vi "Task7_with_case.vi"() -> ()   [LabVIEW 2017]
panel:
  out "String":string
  out "Binary":i8 format="%b"
  out "Decimal":string
  out "Octal":string
  out "Hexadecimal":string
  in  "Array":bool[](array[boolean])
  in  "0 - binary, 1 - octal, 2 - decimal, 3 - hexadecimal":u8(knob) scale=0.0..3.0
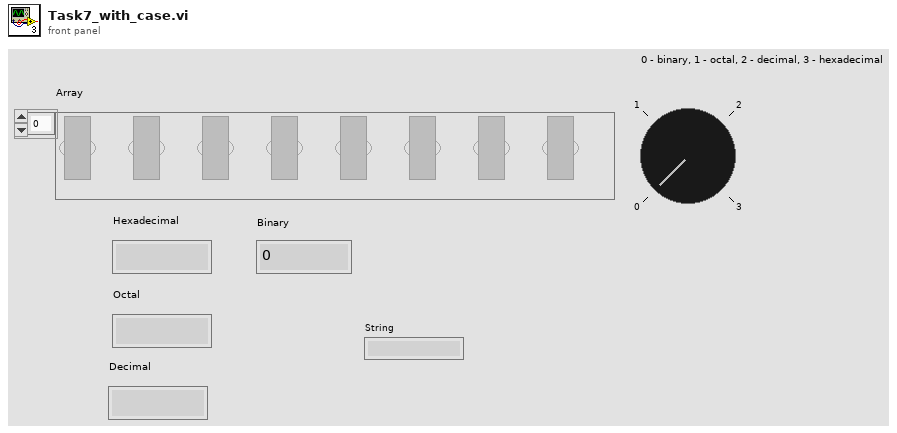
[diagram p1: front panel]
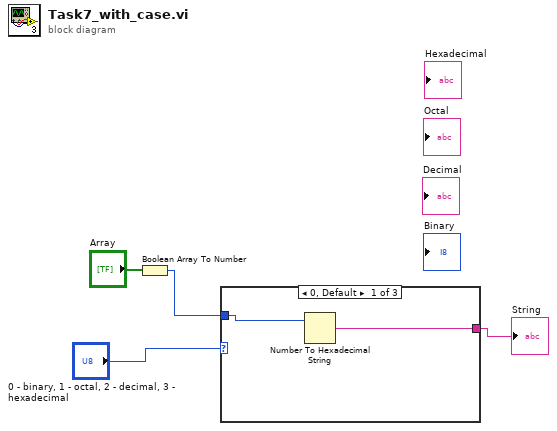
[diagram p0: block diagram]
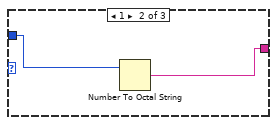
[diagram p2: hidden frame]
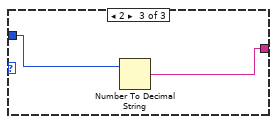
[diagram p3: hidden frame]
diagram:
  n1 = Boolean Array To Number(Boolean array="Array") -> (number=w2:u32)
  n2 = case shown="0, Default" "0 - binary, 1 - octal, 2 - decimal, 3 - hexadecimal" {
    tunnel: w2 -> [w6 w8 w10]
    tunnel: [w5 w7 w9] -> w1
    frame 0, Default {
      n3 = Number To Hexadecimal String(2:w6) -> (0:w5:string)  [unwired: 1 in]
    }
    frame 1 {
      n4 = Number To Octal String(2:w8) -> (0:w7:string)  [unwired: 1 in]
    }
    frame 2 {
      n5 = Number To Decimal String(number=w10) -> (decimal integer string=w9:string)  [unwired: 1 in]
    }
  }
  "String" <- w1
